vi "cwlaserSelectorOpen.vi"   [LabVIEW 2017]
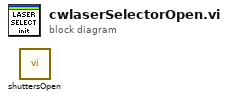
[diagram p0: block diagram]
diagram:
  n1 = call "shuttersOpen.vi"() -> ()  [unwired: 12 in]
